vi "Login Main Panel.vi"(8 "error in (no error)":errorcluster, 11 "User_Actor.lvclass":refnum<class "User_Actor.lvclass">) -> (0 "error out":errorcluster)   [LabVIEW 2015, in "Login.lvclass"]
uses:
  Login.lvclass
  User_Actor/User_Actor/User_Actor.lvclass
  API/_Database/Database.lvclass
  <vilib>/addons/database/Auxilliary.llb/DB Tools Column Info.ctl
  <vilib>/addons/database/Auxilliary.llb/DB Tools DataTypes.ctl
  Login.lvclass/Login.ctl
  <vilib>/Utility/error.llb/Error Cluster From Error Code.vi
  <vilib>/ErrorRing/Error Ring.xnode
  <vilib>/ActorFramework/Actor/Actor.lvclass
  <vilib>/addons/database/NI_Database_API.lvlib
panel:
  in  "Stop":bool
  in  "Register":bool
  in  "Login":bool
  in  "密码":string
  in  "用户名":string
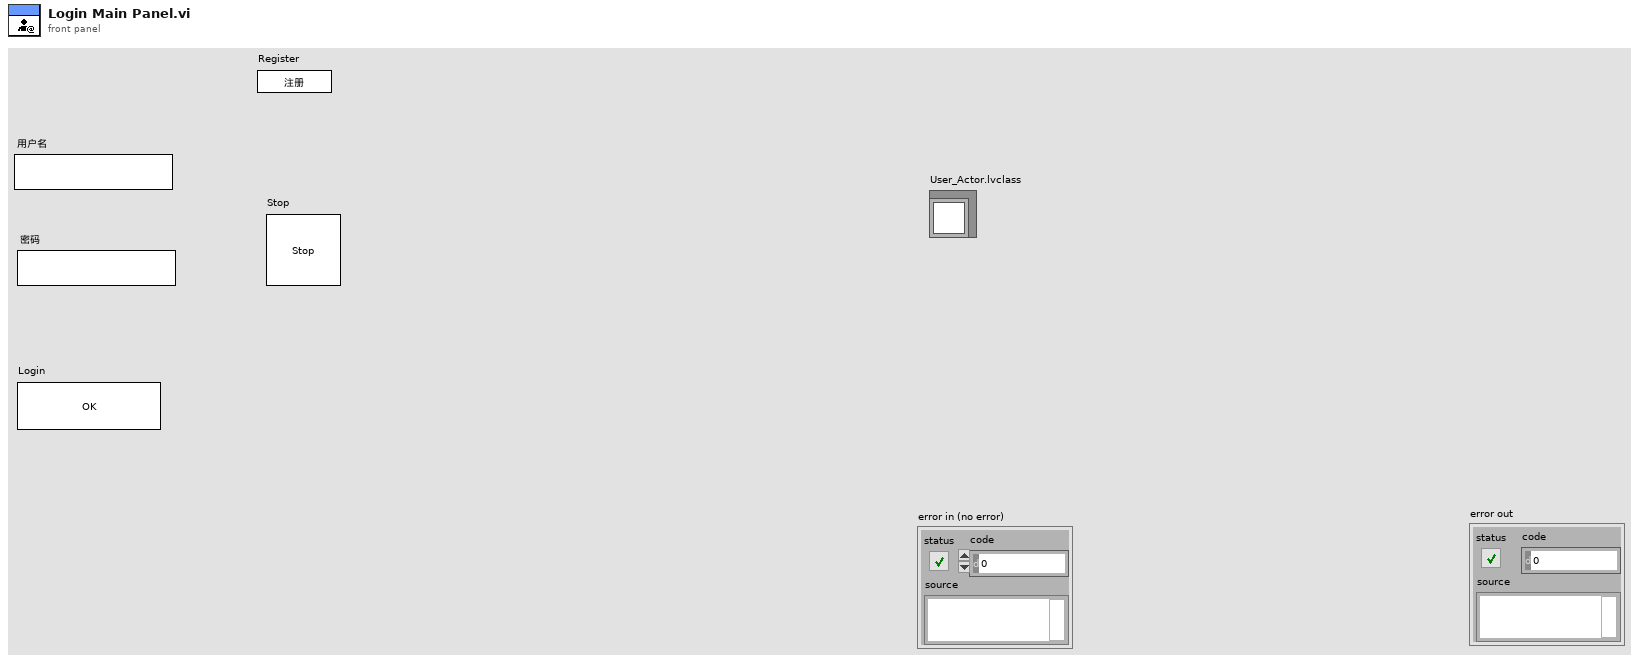
[diagram p1: front panel]
types:
  T1 = typedef "NI_Database_API.lvlib/DB Tools Column Info.ctl" = cluster{"column name":string, "data type":T2, "size":i32, "allow null?":bool}
  T2 = typedef "NI_Database_API.lvlib/DB Tools DataTypes.ctl" = enum16{"String", "Long (I32)", "Single (SGL)", "Double (DBL)", "Date/Time", "Binary"}
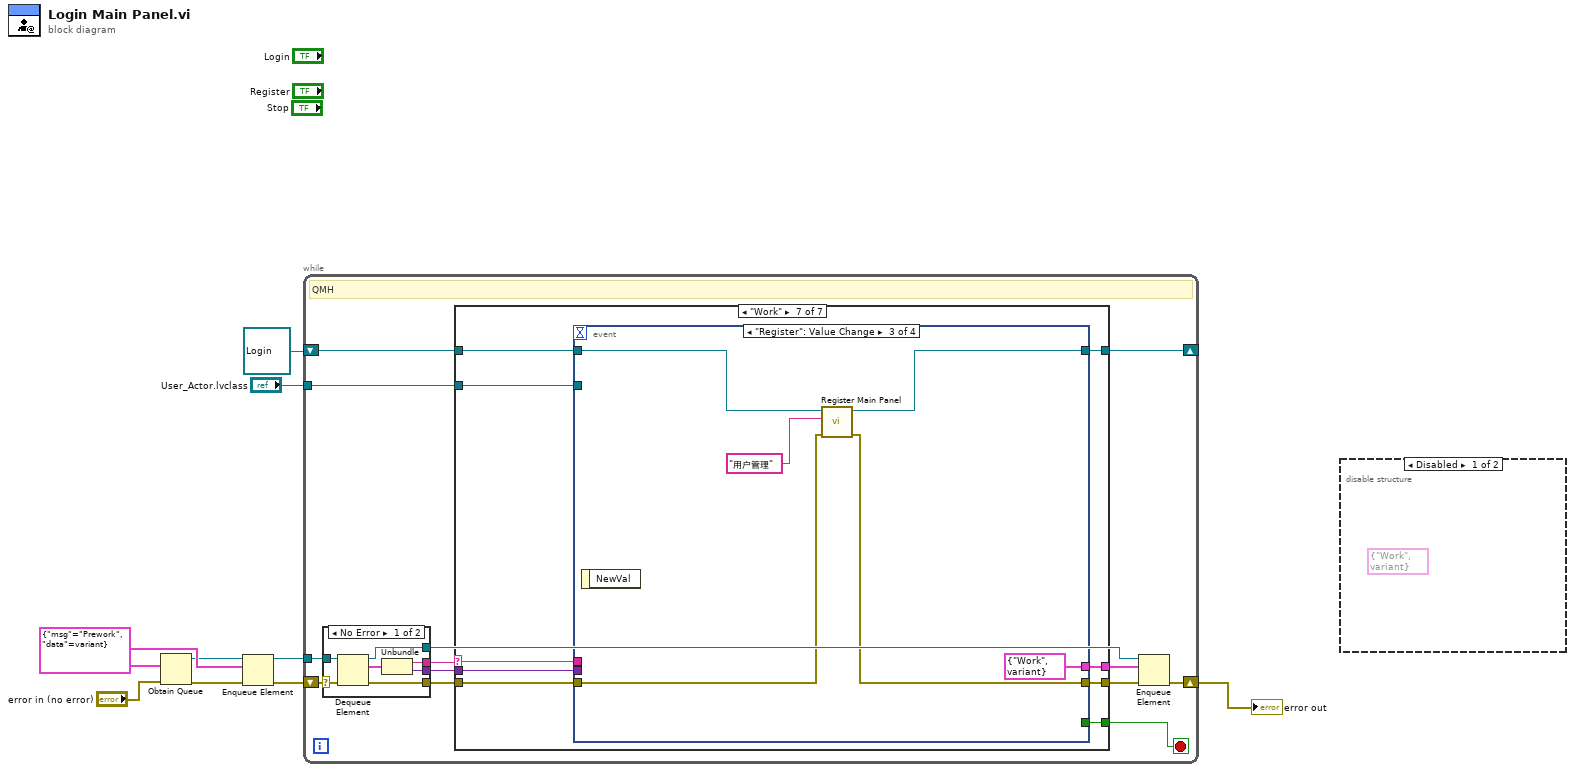
[diagram p0: block diagram]
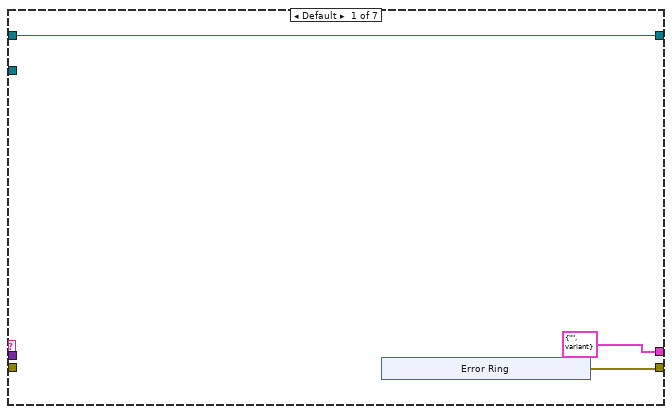
[diagram p3: hidden frame]
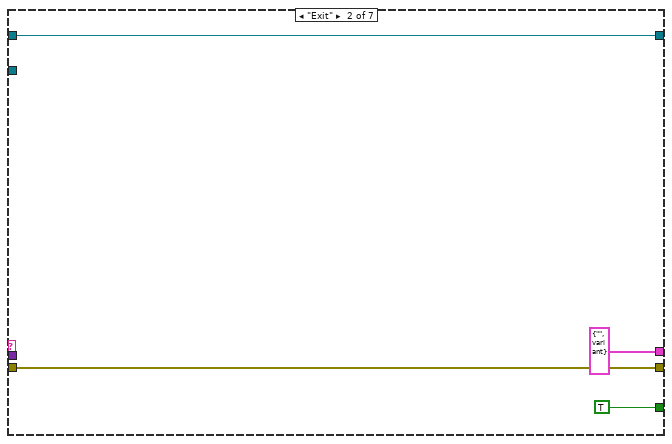
[diagram p4: hidden frame]
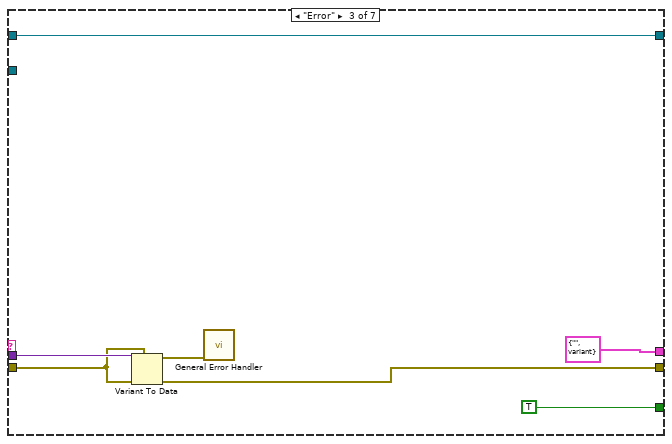
[diagram p5: hidden frame]
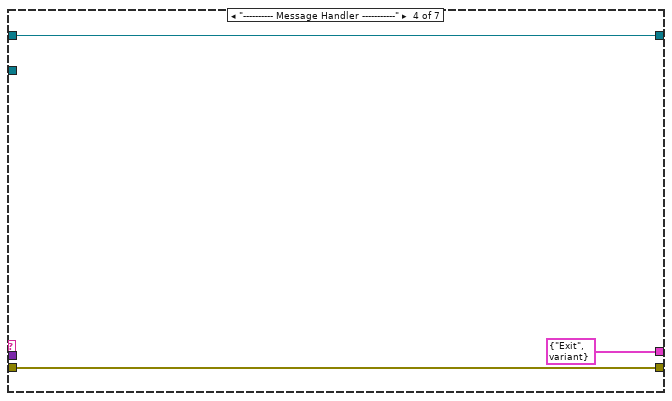
[diagram p6: hidden frame]
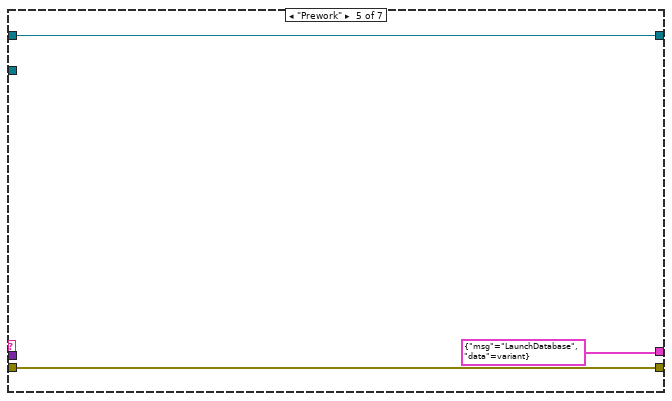
[diagram p7: hidden frame]
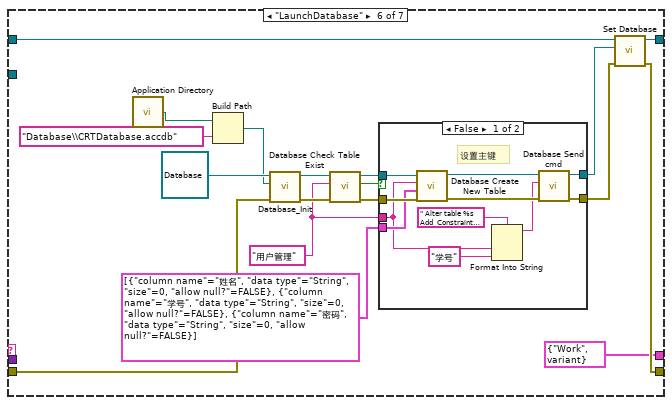
[diagram p8: hidden frame]
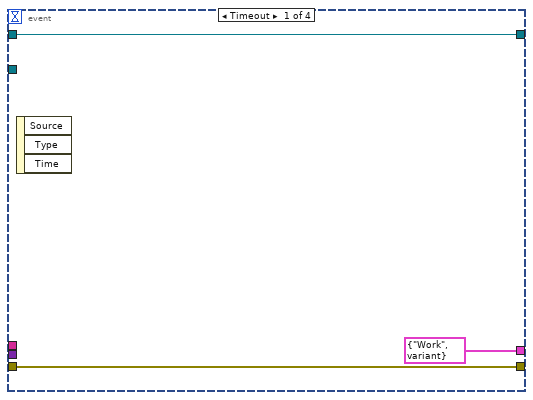
[diagram p10: hidden frame]
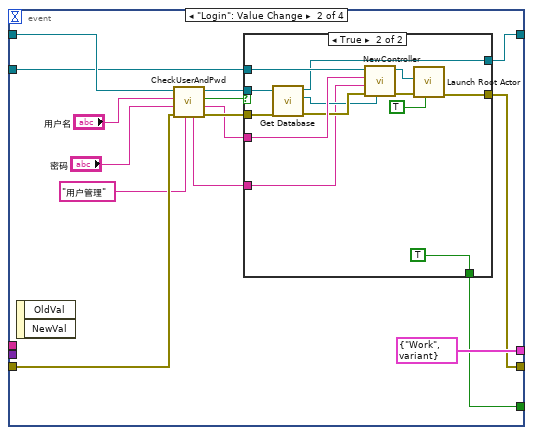
[diagram p11: hidden frame]
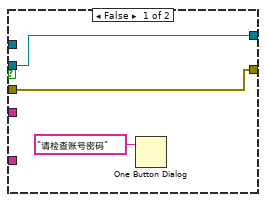
[diagram p12: hidden frame]
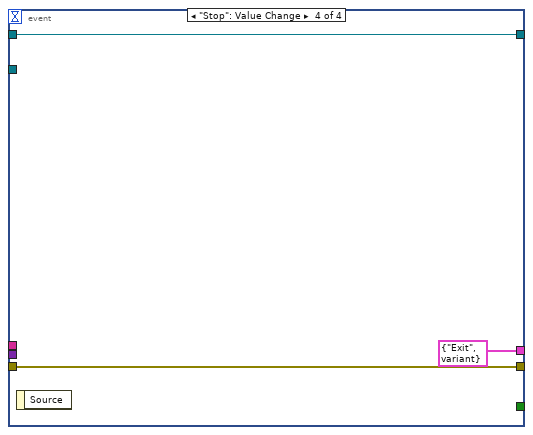
[diagram p13: hidden frame]
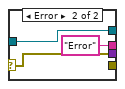
[diagram p14: hidden frame]
diagram:
  w7 = cluster{"msg":string, "data":variant} {"msg"="Prework", "data"=variant}
  n1 = Obtain Queue(element data type=w7, error in (no error)="error in (no error)") -> (queue out=w5:refnum<queue>, error out=w6:errorcluster)  [unwired: 3 in, 1 out]
  n2 = Enqueue Element(queue=w5, element=w7, error in (no error)=w6) -> (queue out=w8:refnum<queue>, error out=w9:errorcluster)  [unwired: 1 in, 1 out]
  n3 = while {
    tunnel: w8 -> [w21]
    shift-right: [w16] -> w1
    shift-left: w9 -> [w22]
    tunnel: "User_Actor.lvclass" -> [w11]
    shift-right: [w10] -> _
    shift-left: refnum<class "Login.lvclass"> refnum ("Login.lvclass") -> [w12]
    stop <- w13 stop-if-true
    # "QMH"
    n4 = case shown="No Error" w22 {
      selector: w22 -> [w136 w140]
      tunnel: w21 -> [w137 w138]
      tunnel: [w135 _] -> w20
      tunnel: [w133 "Error" ("msg")] -> w19
      tunnel: [w132 w140] -> w18
      tunnel: [w131 w138] -> w15
      frame No Error {
        n5 = Dequeue Element(queue=w137, error in (no error)=w136) -> (queue out=w131:refnum<queue>, element=w134:cluster{"msg":string, "data":variant}, error out=w135:errorcluster)  [unwired: 1 in, 1 out]
        n6 = Unbundle(w134) -> ("msg"=w133:string, "data"=w132:variant)
      }
      frame Error {
      }
    }
    n7 = case shown="\"Work\"" w19 {
      selector: w19 -> [_ _ _ _ _ _ w85]
      tunnel: w20 -> [_ w34 w40 w44 w46 w64 w87]
      tunnel: w18 -> [_ _ w41 _ _ _ w86]
      tunnel: [w25 w34 w38 w44 w46 w62 w84] -> w17
      tunnel: [cluster{"msg":string, "data":variant} {"msg"="", "data"=variant} cluster{"msg":string, "data":variant} {"msg"="", "data"=variant} cluster{"msg":string, "data":variant} {"msg"="", "data"=variant} cluster{"msg":string, "data":variant} {"msg"="Exit", "data"=variant} cluster{"msg":string, "data":variant} {"msg"="LaunchDatabase", "data"=variant} cluster{"msg":string, "data":variant} {"msg"="Work", "data"=variant} w83] -> w14
      tunnel: [_ TRUE TRUE _ _ _ w79] -> w13
      tunnel: w12 -> [w23 w31 w35 w42 w45 w63 w82]
      tunnel: w11 -> [_ _ _ _ _ _ w81]
      tunnel: [w23 w31 w35 w42 w45 w61 w80] -> w10
      frame Default {
        n8 = xnode "Error Ring"() -> ("error out"=w25:errorcluster)
      }
      frame "Exit" {
      }
      frame "Error" {
        n9 = Variant To Data(error in=w40, type=w40, Variant=w41) -> (data=w39:errorcluster, error out=w38:errorcluster)
        n10 = call <vilib>:"General Error Handler.vi"("error in (no error)"=w39) -> ()  [unwired: 10 in, 5 out]
      }
      frame "---------- Message Handler -----------" {
      }
      frame "Prework" {
      }
      frame "LaunchDatabase" {
        w54 = "用户管理" ("Table")
        n11 = call <vilib>:"Application Directory.vi"() -> ("Application Directory"=w50:path)
        n12 = Build Path(base path=w50, name or relative path="Database\\CRTDatabase.accdb") -> (appended path=w48:path)
        n13 = call "Database_Init.vi"("error in (no error)"=w64, "path"=w48, "object in"=refnum<class "Database.lvclass"> refnum ("Database")) -> ("error out"=w58:errorcluster, "object out"=w59:refnum<class "Database.lvclass">)  [unwired: 7 in]
        n14 = call "Database Check Table Exist.vi"("error in (no error)"=w58, "Table"=w54, "Database in"=w59) -> ("error out"=w55:errorcluster, "Exit?"=w57:bool, "Database out"=w56:refnum<class "Database.lvclass">)  [unwired: 6 in]
        n15 = case shown="False" w57 {
          tunnel: w56 -> [w76 w78]
          tunnel: w55 -> [w75 w77]
          tunnel: w54 -> [w69 _]
          tunnel: T1[] [{"column name"="姓名", "data type"=enum."String", "size"=0, "allow null?"=FALSE}, {"column name"="学号", "data type"=enum."String", "size"=0, "allow null?"=FALSE}, {"column name"="密码", "data type"=enum."String", "size"=0, "allow null?"=FALSE}] ("column information") -> [w74 _]
          tunnel: [w67 w77] -> w51
          tunnel: [w66 w78] -> w52
          frame False {
            # "设置主键"
            n16 = call "Database Create New Table.vi"("error in (no error)"=w75, "column information"=w74, "table"=w69, "Database in"=w76) -> ("error out"=w72:errorcluster, "Database out"=w73:refnum<class "Database.lvclass">)  [unwired: 6 in]
            n17 = Format Into String(format string=" Alter table %s Add  Constraint  PrimaryKey  Primary  Key (%s)" ("SQL query"), w69, "学号" ("input 2")) -> (resulting string=w68:string)  [unwired: 2 in, 1 out]
            n18 = call "Database Send cmd.vi"("error in (no error)"=w72, "SQL query"=w68, "Database in"=w73) -> ("error out"=w67:errorcluster, "Database out"=w66:refnum<class "Database.lvclass">)  [unwired: 7 in]
          }
          frame True {
          }
        }
        n19 = call "Set Database.vi"("error in (no error)"=w51, "Database"=w52, "Login in"=w63) -> ("error out"=w62:errorcluster, "Login out"=w61:refnum<class "Login.lvclass">)  [unwired: 7 in]
      }
      frame "Work" {
        n20 = event shown="[2] \"Register\": Value Change" {
          selector: _ -> [_ _ _ _]
          dyn-events: _ -> [_ _ _ _]
          timeout: _ -> [_ _ _ _]
          tunnel: w87 -> [w90 w103 w125 w130]
          tunnel: w86 -> [_ _ _ _]
          tunnel: w85 -> [_ _ _ _]
          tunnel: [w90 w94 w124 w130] -> w84
          tunnel: [cluster{"msg":string, "data":variant} {"msg"="Work", "data"=variant} cluster{"msg":string, "data":variant} {"msg"="Work", "data"=variant} cluster{"msg":string, "data":variant} {"msg"="Work", "data"=variant} cluster{"msg":string, "data":variant} {"msg"="Exit", "data"=variant}] -> w83
          tunnel: w82 -> [w88 w105 w127 w128]
          tunnel: w81 -> [_ w97 _ _]
          tunnel: [w88 w93 w123 w128] -> w80
          tunnel: [_ w92 _ _] -> w79
          event Timeout {
            n21 = event-data() -> ()  [unwired: 1 in, 3 out]
          }
          event "Login": Value Change {
            n22 = event-data() -> ()  [unwired: 1 in, 2 out]
            n23 = call "CheckUserAndPwd.vi"("TableName(\"\")"="用户管理" ("TableName(\"\")"), "error in (no error)"=w103, "Pwd(\"\")"="密码", "Name(\"\")"="用户名", "Login in"=w105) -> ("error out"=w99:errorcluster, "ID('')"=w95:string, "Has(False)"=w100:bool, "Login out"=w98:refnum<class "Login.lvclass">, "ActualName(\"\")"=w91:string)  [unwired: 2 in]
            n24 = case shown="True" w100 {
              tunnel: w99 -> [w108 w118]
              tunnel: w98 -> [w107 w119]
              tunnel: w97 -> [_ w121]
              tunnel: w95 -> [_ w120]
              tunnel: [w108 w112] -> w94
              tunnel: [w107 w111] -> w93
              tunnel: [_ TRUE] -> w92
              tunnel: w91 -> [_ w109]
              frame False {
                n25 = One Button Dialog(message="请检查账号密码") -> ()  [unwired: 1 in, 1 out]
              }
              frame True {
                n26 = call "Get Database.vi"("error in (no error)"=w118, "Login in"=w119) -> ("error out"=w117:errorcluster, "Database"=w116:refnum<class "Database.lvclass">, "Login out"=w111:refnum<class "Login.lvclass">)  [unwired: 7 in]
                n27 = call-dynamic "NewController.vi"("Database"=w116, "error in (no error)"=w117, "Name('')"=w109, "ID(\"\")"=w120, "User_Actor in"=w121) -> ("error out"=w114:errorcluster, "User_Actor out"=w115:refnum<class "User_Actor.lvclass">)  [unwired: 5 in]
                n28 = call <vilib>:"Launch Root Actor.vi"("Open Actor Core front panel? (F)"=TRUE, "error in (no error)"=w114, "Actor"=w115) -> ("error out"=w112:errorcluster)  [unwired: 7 in, 1 out]
              }
            }
          }
          event "Register": Value Change {
            n29 = event-data() -> ()  [unwired: 1 in, 1 out]
            n30 = call "Register Main Panel.vi"("error in (no error)"=w125, "TableName"="用户管理", "Login.lvclass"=w127) -> ("error out"=w124:errorcluster, "Login out"=w123:refnum<class "Login.lvclass">)  [unwired: 7 in]
          }
          event "Stop": Value Change {
            n31 = event-data() -> ()  [unwired: 1 in, 1 out]
          }
        }
      }
    }
    n32 = Enqueue Element(queue=w15, element=w14, error in (no error)=w17) -> (error out=w16:errorcluster)  [unwired: 1 in, 2 out]
  }
  "error out" <- w1
  n33 = disable-structure shown="Disabled" {
    frame Disabled {
      (unwired) cluster{"msg":string, "data":variant} {"msg"="Work", "data"=variant}
    }
    frame Enabled {
    }
  }
